vi "SS_DAQ_MAIN_FPGA.vi"(6 "Main Cluster IN":T2, 7 "FPGA Reference IN":T5={"Drop0"={"SS_FPGA_Drop0 Error"={"status"=FALSE, "code"=61003, "source"="niLvFpga_Run_Dynamic.vi"}, "FPGA VI Reference Out"=refnum}, "Drop1"={"SS_FPGA_Drop1 Error"={"status"=FALSE, "code"=61003, "source"="niLvFpga_Run_Dynamic.vi"}, "FPGA VI Reference Out 2"=refnum}}, 8 "Error In":errorcluster, 11 "Info In":string="SS ThermoRec Received Trigger\nPulse Number is 111111\nPulse Type is 4\n\nDuration (s) is  10.000000\nDelay (s)  is  10.000000\nScan Period (ms) is  20\nNumber of Samples is  501\n\nDelay Started\nDelay Complete\nExternal Measurement of Delay (s): 10.000000\n\nACQUIRING DATA") -> (0 "Error Out":errorcluster, 1 "Drop1 Data OUT":fxp[][](array[numeric]), 2 "Drop0 Data OUT":fxp[][](array[numeric]), 3 "Info Out":string, 4 "Main Cluster OUT":T2, 5 "FPGA Reference OUT":T5)   [LabVIEW 2016]
uses:
  Control/Control_Main.ctl
  Control/Control_ModuleArray.ctl
  <vilib>/Utility/error.llb/Error Cluster From Error Code.vi
  <vilib>/rvi/errors/niLvFpgaAdjustHostInterfaceError.vi
  <vilib>/rvi/interface/nirviReadWriteControl/nirviReadWriteControl.xnode
  <vilib>/rvi/interface/nirviMethod/nirviMethod.xnode
  NiFpgaLv.dll
  <vilib>/rvi/interface/Simulation/niFpgaSimulationCallBeginRW.vi
  <vilib>/FPGAPlugInAG/Dynamic/niLvFpga_ReadFifo_Dynamic.vi
  <vilib>/rvi/errors/niLvFpgaMergeErrorWithErrorCode.vi
panel:
  in  "Tab Control":T1(tab)=enum."FPGA Reference"
  out "FPGA Info":T4
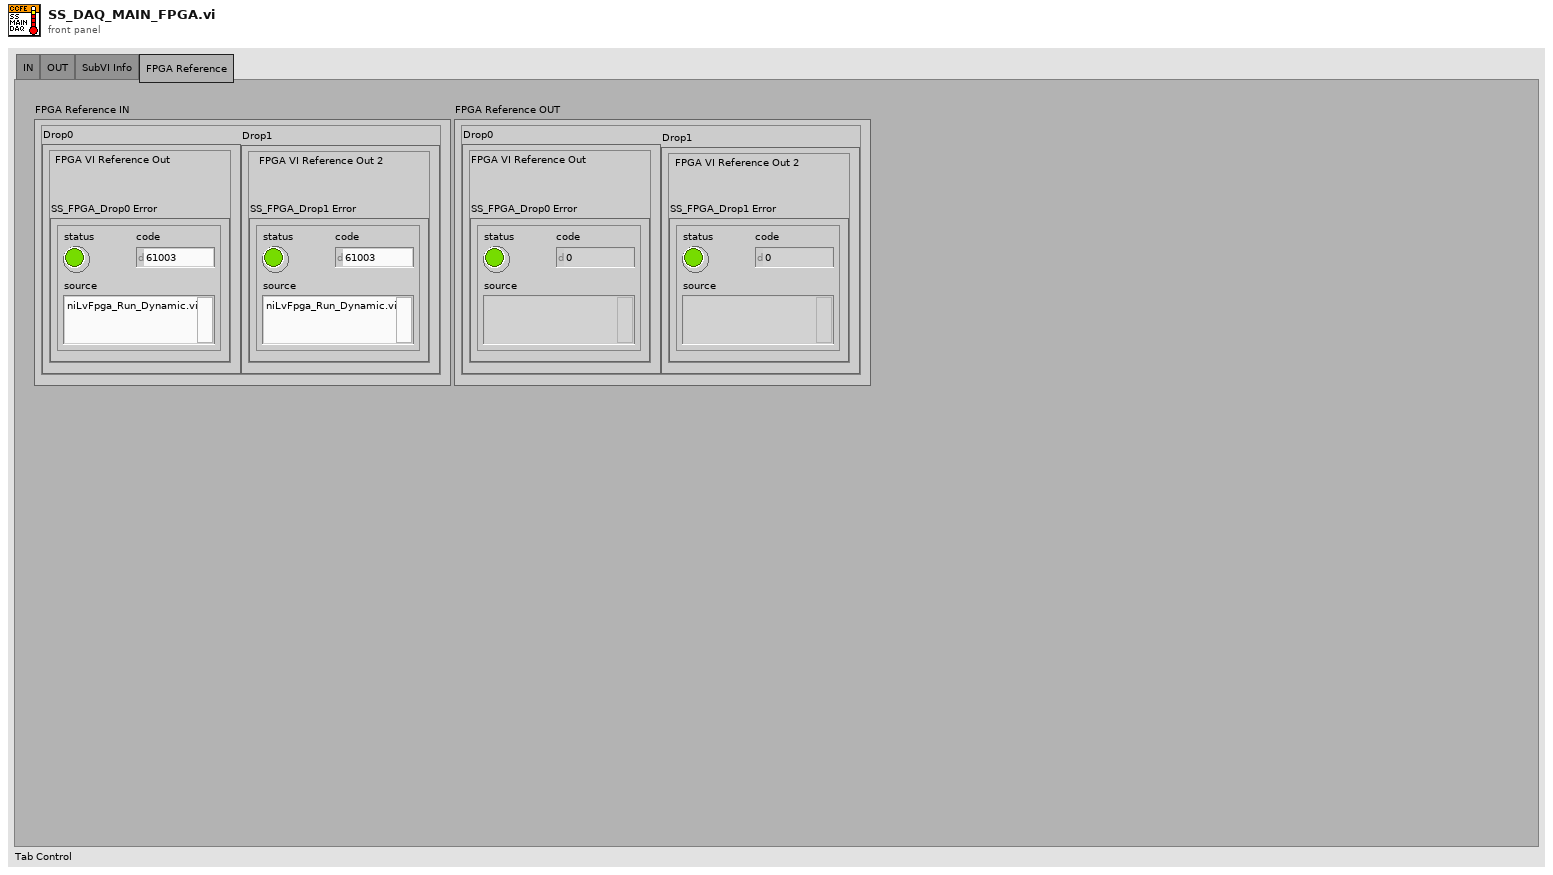
[diagram p1: front panel]
types:
  T1 = enum32{"IN", "OUT", "SubVI Info", "FPGA Reference"}
  T2 = typedef "Control_Main.ctl" = cluster{"Device Cluster":cluster{"Module Array":T3, "Version Number":string, "Version Information":string}, "Input Cluster":cluster{"Input String":string, "Drop1 Target Address":string, "Drop2 Target Address":string, "System":string}, "Data Cluster Out":cluster{"Timing Cluster":cluster{"Number of Samples":i32, "Scan Period (mSec)":u32, "Duration (s)":dbl, "Delay (s)":dbl}, "Time Array":dbl[], "Actual Samples":i32, "Actual Duration":string, "Data Collection Error":bool}, "Path Cluster":cluster{"Full File Name and Path (path)":path, "Full File Name and Path (string)":string}, "File Success Cluster":cluster{"ThermoRec_FileSaved":i32, "File Create Status":bool, "File Error":errorcluster, "File Status":string}, "FTP Success Cluster":cluster{"FTP Success Int":i32, "FTP Success String":string}, "Debug String":string}
  T3 = typedef "Control_ModuleArray.ctl" = cluster{"Drop":i32, "Module":i32, "Module Info":string, "Enabled":bool, "Channel Array":cluster{"ID":i32, "Channel No.":i32, "Enabled":bool, "Channel Name":string, "Channel Info":string, "Units":string, "Scale - M":dbl, "Scale - c":dbl, "Data Array":dbl[]}[]}[]
  T4 = cluster{"Drop0":cluster{"Number of Channels":i32, "Actual Number of Samples":i32, "Actual Duration (ms)":u32, "Duration (mSec)":u32, "Complete":bool, "Start Acquisition":bool, "Scan Rate (mSec)":u32, "Error Out":errorcluster, "Elements Remaining":u32}, "Drop1":cluster{"Number of Channels":i32, "Actual Number of Samples":i32, "Actual Duration (ms)":u32, "Duration (mSec)":u32, "Complete":bool, "Start Acquisition":bool, "Scan Rate (mSec)":u32, "Error Out":errorcluster, "Elements Remaining":u32}}
  T5 = cluster{"Drop0":cluster{"SS_FPGA_Drop0 Error":errorcluster, "FPGA VI Reference Out":refnum<k20>}, "Drop1":cluster{"SS_FPGA_Drop1 Error":errorcluster, "FPGA VI Reference Out 2":refnum<k20>}}
  T6 = cluster{"Drop0":cluster{"Actual Duration (ms)":i32, "Actual Number of Samples":i32}, "Drop1":cluster{"Actual Duration (ms)":i32, "Actual Number of Samples":i32}}
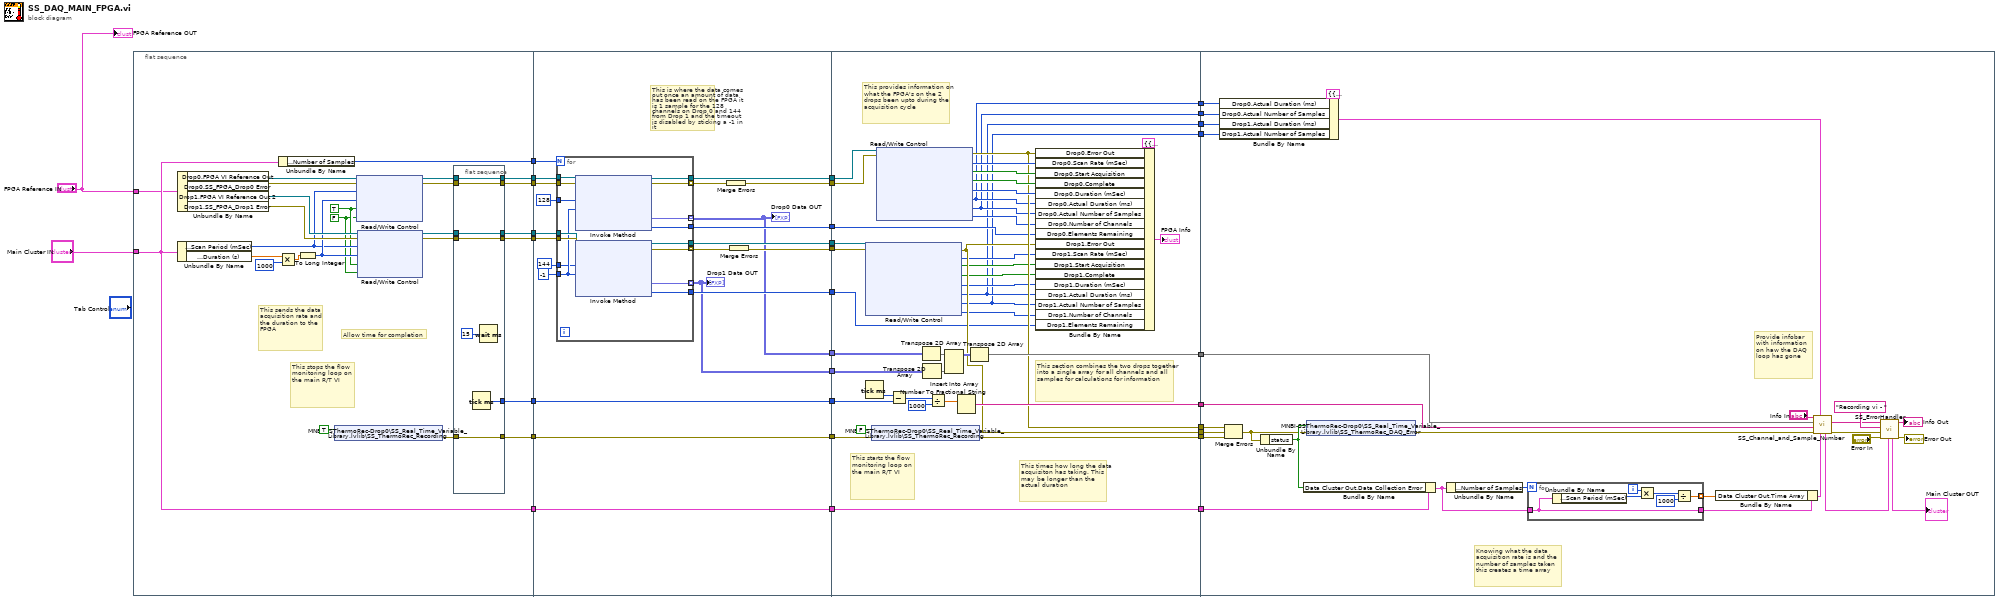
[diagram p0: block diagram]
diagram:
  n1 = flat-sequence {
    tunnel: "FPGA Reference IN" -> [w33]
    tunnel: "Main Cluster IN" -> [w34]
    tunnel: [w40] -> w31
    tunnel: [w39] -> w30
    tunnel: [w38] -> w29
    tunnel: [w37] -> w28
    tunnel: [w36] -> w27
    tunnel: [w34] -> w25
    tunnel: [w35] -> w24
    tunnel: [w32] -> w15
    tunnel: [w76] -> w23
    tunnel: [w74] -> w22
    tunnel: w31 -> [w77]
    tunnel: w30 -> [w79]
    tunnel: w29 -> [w80]
    tunnel: w28 -> [w78]
    tunnel: [w75] -> w21
    tunnel: [w73] -> w20
    tunnel: [w68] -> w19
    tunnel: w27 -> [w68]
    tunnel: w25 -> [w85]
    tunnel: [w85] -> w18
    tunnel: w24 -> [w81]
    tunnel: [w69] -> w17
    tunnel: [w70] -> w16
    tunnel: w15 -> [w67]
    tunnel: [w67] -> w14
    tunnel: [w66] -> w13
    tunnel: [w65] -> w12
    tunnel: w23 -> [w140]
    tunnel: w21 -> [w139]
    tunnel: w22 -> [w138]
    tunnel: w20 -> [w137]
    tunnel: w18 -> [w127]
    tunnel: w17 -> [w112]
    tunnel: w16 -> [w105]
    tunnel: w19 -> [w135]
    tunnel: w14 -> [w132]
    tunnel: w13 -> [w129]
    tunnel: w12 -> [w128]
    tunnel: [w127] -> w11
    tunnel: [w125] -> w10
    tunnel: [w123] -> w9
    tunnel: [w122] -> w8
    tunnel: [w111] -> w7
    tunnel: [w114] -> w6
    tunnel: [w104] -> w4
    tunnel: [w103] -> w3
    tunnel: [w102] -> w2
    tunnel: [w101] -> w1
    tunnel: w11 -> [w151]
    tunnel: w10 -> [w142]
    tunnel: w9 -> [w143]
    tunnel: w8 -> [w152]
    tunnel: w7 -> [w153]
    tunnel: w6 -> [w154]
    tunnel: w4 -> [w149]
    tunnel: w3 -> [w148]
    tunnel: w2 -> [w147]
    tunnel: w1 -> [w146]
    frame #0 {
      w46 = FALSE
      w47 = TRUE
      # "This stops the flow monitoring loop on the main R/T VI"
      # "This sends the data acquisition rate and the duration to the FPGA"
      # "Allow time for completion"
      n2 = Unbundle By Name(w34) -> ("Data Cluster Out.Timing Cluster.Scan Period (mSec)"=w48:u32, "Data Cluster Out.Timing Cluster.Duration (s)"=w52:dbl)
      n3 = Unbundle By Name(w33) -> ("Drop0.FPGA VI Reference Out"=w56:refnum<k20>, "Drop0.SS_FPGA_Drop0 Error"=w55:errorcluster, "Drop1.FPGA VI Reference Out 2"=w53:refnum<k20>, "Drop1.SS_FPGA_Drop1 Error"=w54:errorcluster)
      n4 = Unbundle By Name(w34) -> ("Data Cluster Out.Timing Cluster.Number of Samples"=w35:i32)
      n5 = Multiply(x=w52, y=1000) -> (x*y=w50:dbl)
      n6 = To Long Integer(number=w50) -> (32bit integer=w49:i32)
      n7 = shared-variable "MNBI-SSThermoRec-Drop0\\SS_Real_Time_Variable_Library.lvlib\\SS_ThermoRec_Recording"(TRUE ("SS_ThermoRec_Recording")) -> (error out=w41:errorcluster)  [unwired: 1 in]
      n8 = xnode "Read/Write Control"("FPGA VI Reference In"=w56, "error in"=w55, "Scan Rate (mSec)"=w48, "Duration (mSec)"=w49, "Start Acquisition"=w47, "Complete"=w46) -> ("FPGA VI Reference Out"=w45:refnum<k20>, "error out"=w43:errorcluster)
      n9 = xnode "Read/Write Control"("FPGA VI Reference In"=w53, "error in"=w54, "Scan Rate (mSec)"=w48, "Duration (mSec)"=w49, "Start Acquisition"=w47, "Complete"=w46) -> ("FPGA VI Reference Out"=w44:refnum<k20>, "error out"=w42:errorcluster)
      n10 = flat-sequence {
        tunnel: w45 -> [w64]
        tunnel: w44 -> [w63]
        tunnel: [w64] -> w40
        tunnel: [w63] -> w39
        tunnel: w43 -> [w61]
        tunnel: w42 -> [w60]
        tunnel: w41 -> [w59]
        tunnel: [w61] -> w38
        tunnel: [w60] -> w37
        tunnel: [w59] -> w36
        tunnel: [w58] -> w32
        frame #0 {
          n11 = Tick Count (ms)() -> (millisecond timer value=w58:u32)
          n12 = Wait (ms)(milliseconds to wait=u32 15) -> ()  [unwired: 1 out]
        }
      }
    }
    frame #1 {
      # "This is where the data comes out once an amount of data has been read on the FPGA it is 1 sample for the 128 channels on Drop 0 and 144 from Drop 1 and the timeout is disabled by sticking a -1 in it"
      n13 = for {
        N: w81 -> [_]
        tunnel: -1 -> [w95]
        tunnel: [w91] -> w65 mode=indexing
        tunnel: [w94] -> w66 mode=indexing
        tunnel: [w99] -> w76
        tunnel: [w98] -> w83 mode=indexing
        tunnel: [w93] -> w74
        tunnel: [w92] -> w84 mode=indexing
        tunnel: w78 -> [w97]
        tunnel: w79 -> [w96]
        tunnel: w80 -> [w100]
        tunnel: w77 -> [w90]
        tunnel: 128 -> [w89]
        tunnel: 144 -> [w88]
        tunnel: [w87] -> w70
        tunnel: [w86] -> w69
        n14 = xnode "Invoke Method"("FPGA VI Reference In"=w96, "error in"=w97, "Number of Elements"=w88, "Timeout (ms)"=w95) -> ("FPGA VI Reference Out"=w93:refnum<k20>, "error out"=w92:errorcluster, "Data"=w91:fxp<+/-,15,14>[], "Elements Remaining"=w87:u32)
        n15 = xnode "Invoke Method"("FPGA VI Reference In"=w90, "error in"=w100, "Number of Elements"=w89, "Timeout (ms)"=w95) -> ("FPGA VI Reference Out"=w99:refnum<k20>, "error out"=w98:errorcluster, "Data"=w94:fxp<+/-,15,14>[], "Elements Remaining"=w86:u32)
      }
      "Drop0 Data OUT" <- w66
      "Drop1 Data OUT" <- w65
      n16 = Merge Errors(w83) -> (w75:errorcluster)
      n17 = Merge Errors(w84) -> (w73:errorcluster)
    }
    frame #2 {
      # "This starts the flow monitoring loop on the main R/T VI"
      # "This provides information on what the FPGA's on the 2 drops been upto during the acquisition cycle"
      # "This times how long the data acquisiton has taking. This may be longer than the actual duration"
      # "This section combines the two drops together into a single array for all channels and all samples for calculations for information"
      n18 = Tick Count (ms)() -> (millisecond timer value=w131:u32)
      n19 = xnode "Read/Write Control"("FPGA VI Reference In"=w138, "error in"=w137) -> ("error out"=w111:errorcluster, "Scan Rate (mSec)"=w110:u32, "Start Acquisition"=w109:bool, "Complete"=w108:bool, "Duration (mSec)"=w107:u32, "Actual Duration (ms)"=w102:u32, "Actual Number of Samples"=w101:i32, "Number of Channels"=w106:i32)  [unwired: 1 out]
      n20 = shared-variable "MNBI-SSThermoRec-Drop0\\SS_Real_Time_Variable_Library.lvlib\\SS_ThermoRec_Recording"(FALSE ("SS_ThermoRec_Recording"), error in=w135) -> (error out=w122:errorcluster)
      n21 = xnode "Read/Write Control"("FPGA VI Reference In"=w140, "error in"=w139) -> ("error out"=w114:errorcluster, "Scan Rate (mSec)"=w118:u32, "Start Acquisition"=w117:bool, "Complete"=w116:bool, "Duration (mSec)"=w115:u32, "Actual Duration (ms)"=w104:u32, "Actual Number of Samples"=w103:i32, "Number of Channels"=w113:i32)  [unwired: 1 out]
      n22 = Subtract(x=w131, y=w132) -> (x-y=w134:u32)
      n23 = Transpose 2D Array(2D array=w129) -> (transposed array=w130:fxp<+/-,15,14>[][])
      n24 = Transpose 2D Array(2D array=w128) -> (transposed array=w121:fxp<+/-,15,14>[][])
      n25 = Divide(x=w134, y=u32 1000) -> (x/y=w126:dbl)
      n26 = Insert Into Array(array=w130, new element=w121) -> (w124:fxp<+/-,15,14>[][])  [unwired: 2 in]
      n27 = Number To Fractional String(number=w126) -> (F-format string=w125:string)  [unwired: 3 in]
      n28 = Transpose 2D Array(2D array=w124) -> (transposed array=w123:fxp<+/-,15,14>[][])
      n29 = Bundle By Name(cluster=T4 {"Drop0"={"Number of Channels"=0, "Actual Number of Samples"=0, "Actual Duration (ms)"=0, "Duration (mSec)"=0, "Complete"=FALSE, "Start Acquisition"=FALSE, "Scan Rate (mSec)"=0, "Error Out"={"status"=FALSE, "code"=0, "source"=""}, "Elements Remaining"=0}, "Drop1"={"Number of Channels"=0, "Actual Number of Samples"=0, "Actual Duration (ms)"=0, "Duration (mSec)"=0, "Complete"=FALSE, "Start Acquisition"=FALSE, "Scan Rate (mSec)"=0, "Error Out"={"status"=FALSE, "code"=0, "source"=""}, "Elements Remaining"=0}} ("FPGA Info 2"), "Drop0.Error Out"=w114, "Drop0.Scan Rate (mSec)"=w118, "Drop0.Start Acquisition"=w117, "Drop0.Complete"=w116, "Drop0.Duration (mSec)"=w115, "Drop0.Actual Duration (ms)"=w104, "Drop0.Actual Number of Samples"=w103, "Drop0.Number of Channels"=w113, "Drop0.Elements Remaining"=w112, "Drop1.Error Out"=w111, "Drop1.Scan Rate (mSec)"=w110, "Drop1.Start Acquisition"=w109, "Drop1.Complete"=w108, "Drop1.Duration (mSec)"=w107, "Drop1.Actual Duration (ms)"=w102, "Drop1.Actual Number of Samples"=w101, "Drop1.Number of Channels"=w106, "Drop1.Elements Remaining"=w105) -> (→"FPGA Info":T4)
    }
    frame #3 {
      # "Provide infobar with information on haw the DAQ loop has gone"
      # "Knowing what the data acquisition rate is and the number of samples taken this creates a time array"
      n30 = Bundle By Name(cluster=T6 {"Drop0"={"Actual Duration (ms)"=0, "Actual Number of Samples"=0}, "Drop1"={"Actual Duration (ms)"=0, "Actual Number of Samples"=0}} ("FPGA Info IN"), "Drop0.Actual Duration (ms)"=w149, "Drop0.Actual Number of Samples"=w148, "Drop1.Actual Duration (ms)"=w147, "Drop1.Actual Number of Samples"=w146) -> (w141:T6)
      n31 = Merge Errors(w154, w153, w152) -> (w155:errorcluster)
      n32 = Unbundle By Name(w155) -> ("status"=w158:bool)
      n33 = Bundle By Name(cluster=w151, "Data Cluster Out.Data Collection Error"=w158) -> (w157:T2)
      n34 = shared-variable "MNBI-SSThermoRec-Drop0\\SS_Real_Time_Variable_Library.lvlib\\SS_ThermoRec_DAQ_Error"(w158, error in=w155) -> (error out=w144:errorcluster)
      n35 = Unbundle By Name(w157) -> ("Data Cluster Out.Timing Cluster.Number of Samples"=w160:i32)
      n36 = for {
        N: w160 -> [_]
        tunnel: [w175] -> w159
        tunnel: w157 -> [w175]
        tunnel: [w171] -> w156 mode=indexing
        i -> [w174]
        n37 = Unbundle By Name(w175) -> ("Data Cluster Out.Timing Cluster.Scan Period (mSec)"=w170:u32)
        n38 = Multiply(x=w174, y=w170) -> (x*y=w173:u32)
        n39 = Divide(x=w173, y=u32 1000) -> (x/y=w171:dbl)
      }
      n40 = Bundle By Name(cluster=w159, "Data Cluster Out.Time Array"=w156) -> (w145:T2)
      n41 = call "SS_Channel_and_Sample_Number.vi"("Main Cluster IN"=w145, "FPGA Info IN"=w141, "Error In"=w144, "RT Duration"=w142, "DATA"=w143, "Info In"="Info In") -> ("Error Out"=w164:errorcluster, "Info Out"=w162:string, "Main Cluster OUT"=w163:T2)  [unwired: 3 in]
      n42 = call "SS_ErrorHandler.vi"("Main Cluster IN"=w163, "Error In"="Error In", "SubVI Error"=w164, "SubVI Name"="Recording vi - ", "Info In"=w162) -> ("Error Out"=→"Error Out":errorcluster, "Info Out"=→"Info Out":string, "Main Cluster OUT"=→"Main Cluster OUT":T2)  [unwired: 4 in]
    }
  }
  "FPGA Reference OUT" <- "FPGA Reference IN"
